vi "Read and Sort Inventory.vi"() -> (0 "Array":T1[](array[typedef]))   [LabVIEW 2013]
uses:
  Controls/Display Component Line.ctl
  Controls/Components.ctl
  Controls/Component Sub Type.ctl
  Controls/Add Button.ctl
  Controls/Subtract Button.ctl
  Globals/Inventory Path Global.vi
  <vilib>/Utility/file.llb/Read From Spreadsheet File (string).vi
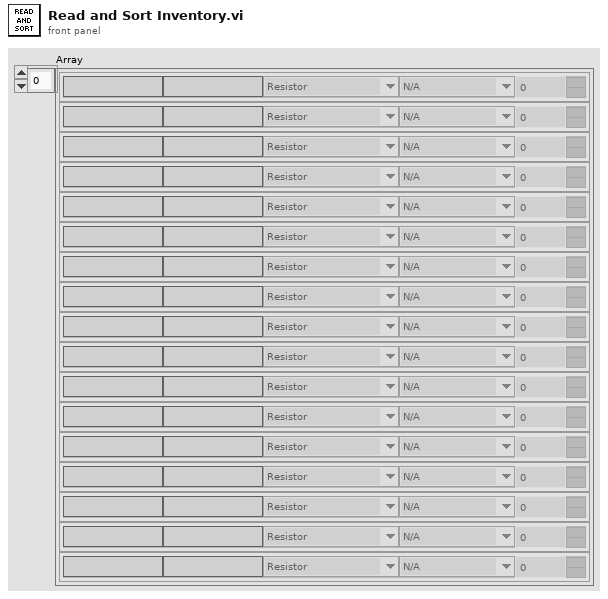
[diagram p1: front panel]
types:
  T1 = typedef "Display Component Line.ctl" = cluster{"Part Number":string, "Code (Value)":string, "Component Type":T2, "Component Subtype":T3, "Quantity":u32, "Add":T4, "Subtract":T5}
  T2 = typedef "Components.ctl" = enum16{"Resistor", "Capacitor", "Diode", "Voltage Regulator", "Transistors", "ICs", "Misc"}
  T3 = typedef "Component Sub Type.ctl" = enum16{"N/A", "Carbon", "Variable - Trimmer", "Variable - Pot", "Ceramic", "Electrolitic", "Zenner", "TO-92", "TO-220", "NPN", "PNP", "CMOS", "Processor"}
  T4 = typedef "Add Button.ctl" = bool
  T5 = typedef "Subtract Button.ctl" = bool
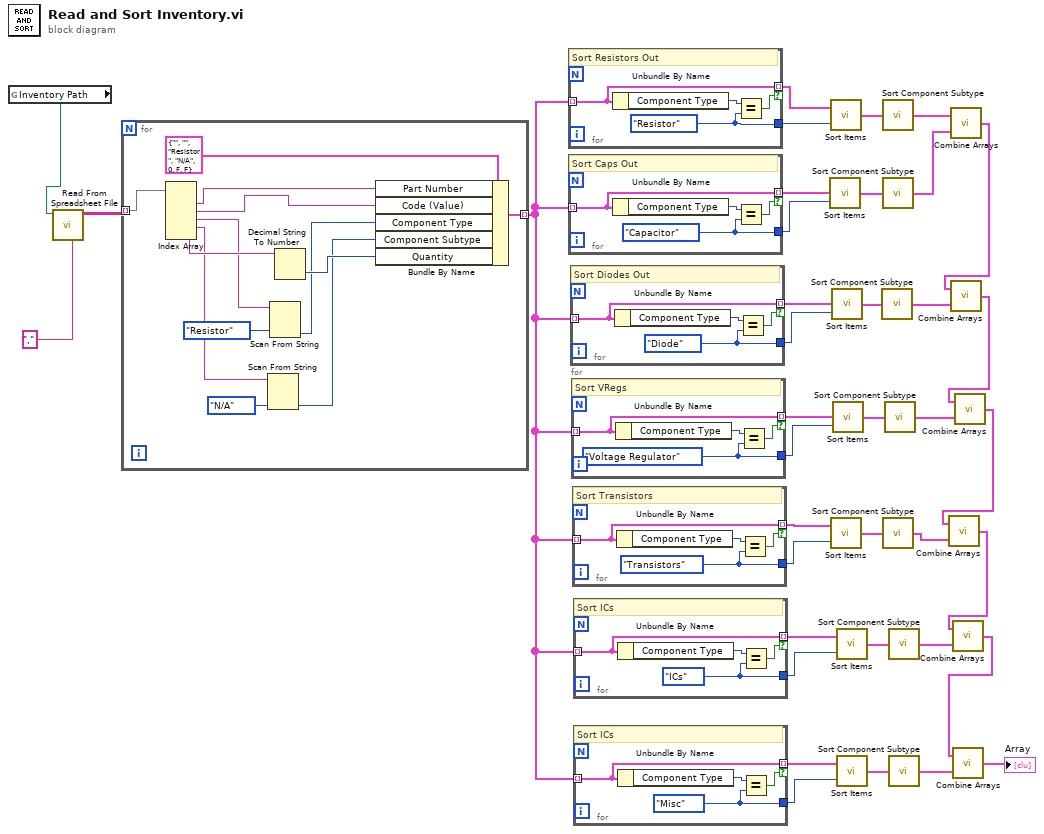
[diagram p0: block diagram]
diagram:
  n1 = global read "Inventory Path Global.vi" "Inventory Path"() -> (w38:path)
  n2 = call-poly <vilib>:"Read From Spreadsheet File.vi"("delimiter (\\t)"="," ("delimiter (\\t)"), "file path (dialog if empty)"=w38) -> ("all rows"=w37:string[][])  [unwired: 5 in, 4 out]
  n3 = for {
    tunnel: w37 -> [w51] mode=indexing
    tunnel: [w47] -> w1 mode=indexing
    n4 = Index Array(array=w51) -> (element #1=w48:string, element #2=w49:string, element #3=w41:string, element #4=w43:string, element #5=w45:string)  [unwired: 5 in]
    n5 = Scan From String(input string=w43, default 1=Component_Sub_Type."N/A" ("Component Subtype")) -> (output 1=w42:T3)  [unwired: 3 in, 3 out]
    n6 = Scan From String(input string=w41, default 1=Components."Resistor" ("Component Type")) -> (output 1=w39:T2)  [unwired: 3 in, 3 out]
    n7 = Decimal String To Number(string=w45) -> (number=w46:i32)  [unwired: 2 in, 1 out]
    n8 = Bundle By Name(cluster=T1 {"Part Number"="", "Code (Value)"="", "Component Type"=enum."Resistor", "Component Subtype"=enum."N/A", "Quantity"=0, "Add"=FALSE, "Subtract"=FALSE} ("Display Components Line"), "Part Number"=w48, "Code (Value)"=w49, "Component Type"=w39, "Component Subtype"=w42, "Quantity"=w46) -> (w47:T1)
  }
  n9 = for {
    tunnel: w1 -> [w54] mode=indexing
    tunnel: [w54] -> w35 mode=indexing if=w53
    tunnel: [w52] -> w34
    w52 = Components."Resistor" ("Component Type")
    # "Sort Resistors Out"
    n10 = Unbundle By Name(w54) -> ("Component Type"=w55:T2)
    n11 = Equal?(x=w55, y=w52) -> (x = y?=w53:bool)
  }
  n12 = for {
    tunnel: w1 -> [w58] mode=indexing
    tunnel: [w58] -> w33 mode=indexing if=w57
    tunnel: [w56] -> w32
    w56 = Components."Capacitor" ("Component Type")
    # "Sort Caps Out"
    n13 = Unbundle By Name(w58) -> ("Component Type"=w59:T2)
    n14 = Equal?(x=w59, y=w56) -> (x = y?=w57:bool)
  }
  n15 = for {
    tunnel: w1 -> [w62] mode=indexing
    tunnel: [w62] -> w28 mode=indexing if=w61
    tunnel: [w60] -> w29
    w60 = Components."Diode" ("Component Type")
    # "Sort Diodes Out"
    n16 = Unbundle By Name(w62) -> ("Component Type"=w63:T2)
    n17 = Equal?(x=w63, y=w60) -> (x = y?=w61:bool)
  }
  n18 = for {
    tunnel: w1 -> [w66] mode=indexing
    tunnel: [w66] -> w27 mode=indexing if=w65
    tunnel: [w64] -> w26
    w64 = Components."Voltage Regulator" ("Component Type")
    # "Sort VRegs"
    n19 = Unbundle By Name(w66) -> ("Component Type"=w67:T2)
    n20 = Equal?(x=w67, y=w64) -> (x = y?=w65:bool)
  }
  n21 = for {
    tunnel: w1 -> [w70] mode=indexing
    tunnel: [w70] -> w19 mode=indexing if=w69
    tunnel: [w68] -> w18
    w68 = Components."Transistors" ("Component Type")
    # "Sort Transistors"
    n22 = Unbundle By Name(w70) -> ("Component Type"=w71:T2)
    n23 = Equal?(x=w71, y=w68) -> (x = y?=w69:bool)
  }
  n24 = for {
    tunnel: w1 -> [w74] mode=indexing
    tunnel: [w74] -> w20 mode=indexing if=w73
    tunnel: [w72] -> w21
    w72 = Components."ICs" ("Component Type")
    # "Sort ICs"
    n25 = Unbundle By Name(w74) -> ("Component Type"=w75:T2)
    n26 = Equal?(x=w75, y=w72) -> (x = y?=w73:bool)
  }
  n27 = for {
    tunnel: w1 -> [w78] mode=indexing
    tunnel: [w78] -> w6 mode=indexing if=w77
    tunnel: [w76] -> w5
    w76 = Components."Misc" ("Component Type")
    # "Sort ICs"
    n28 = Unbundle By Name(w78) -> ("Component Type"=w79:T2)
    n29 = Equal?(x=w79, y=w76) -> (x = y?=w77:bool)
  }
  n30 = call "Sort Items.vi"("Component Type"=w32, "Unsorted Componet In"=w33) -> ("Sorted Component Array Out"=w31:T1[])
  n31 = call "Sort Items.vi"("Component Type"=w34, "Unsorted Componet In"=w35) -> ("Sorted Component Array Out"=w17:T1[])
  n32 = call "Sort Items.vi"("Component Type"=w18, "Unsorted Componet In"=w19) -> ("Sorted Component Array Out"=w23:T1[])
  n33 = call "Sort Items.vi"("Component Type"=w29, "Unsorted Componet In"=w28) -> ("Sorted Component Array Out"=w25:T1[])
  n34 = call "Sort Items.vi"("Component Type"=w26, "Unsorted Componet In"=w27) -> ("Sorted Component Array Out"=w24:T1[])
  n35 = call "Sort Items.vi"("Component Type"=w21, "Unsorted Componet In"=w20) -> ("Sorted Component Array Out"=w22:T1[])
  n36 = call "Sort Items.vi"("Component Type"=w5, "Unsorted Componet In"=w6) -> ("Sorted Component Array Out"=w4:T1[])
  n37 = call "Sort Component Subtype.vi"("Array In"=w25) -> ("Array Out"=w14:T1[])
  n38 = call "Sort Component Subtype.vi"("Array In"=w17) -> ("Array Out"=w16:T1[])
  n39 = call "Sort Component Subtype.vi"("Array In"=w31) -> ("Array Out"=w30:T1[])
  n40 = call "Sort Component Subtype.vi"("Array In"=w23) -> ("Array Out"=w11:T1[])
  n41 = call "Sort Component Subtype.vi"("Array In"=w24) -> ("Array Out"=w12:T1[])
  n42 = call "Sort Component Subtype.vi"("Array In"=w22) -> ("Array Out"=w9:T1[])
  n43 = call "Sort Component Subtype.vi"("Array In"=w4) -> ("Array Out"=w7:T1[])
  n44 = call "Combine Arrays.vi"("Array B In"=w30, "Array A In"=w16) -> ("Array Out"=w15:T1[])
  n45 = call "Combine Arrays.vi"("Array B In"=w14, "Array A In"=w15) -> ("Array Out"=w13:T1[])
  n46 = call "Combine Arrays.vi"("Array B In"=w12, "Array A In"=w13) -> ("Array Out"=w10:T1[])
  n47 = call "Combine Arrays.vi"("Array B In"=w11, "Array A In"=w10) -> ("Array Out"=w8:T1[])
  n48 = call "Combine Arrays.vi"("Array B In"=w9, "Array A In"=w8) -> ("Array Out"=w3:T1[])
  n49 = call "Combine Arrays.vi"("Array B In"=w7, "Array A In"=w3) -> ("Array Out"=→"Array":T1[])
